vi "General Periodic Sinc.vi"(5 "X":dbl[](array[numeric]), 7 "n":i32, 8 "delta t":dbl, 9 "delay":dbl, 10 "amplitude":dbl, 11 "samples":i32) -> (0 "error":i32, 3 "Periodic Sinc Pattern":dbl[](array[numeric]))   [LabVIEW 2014, in "NI_AALBase.lvlib"]
uses:
  NI_AALBase.lvlib
  lvanlys.dll
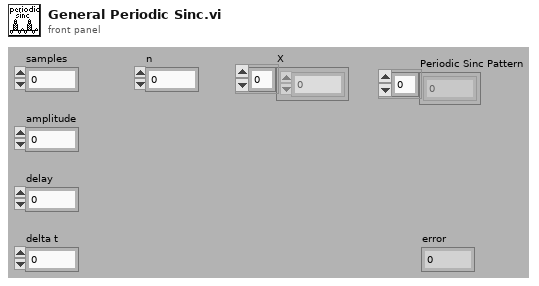
[diagram p1: front panel]
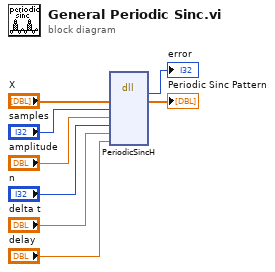
[diagram p0: block diagram]
diagram:
  n1 = dll-call lib="C:/Program Files (x86)/National Instruments/LabVIEW 2014/resource/lvanlys.*" fn="PeriodicSincH"("x"="X", "samples"="samples", "amplitude"="amplitude", "N"="n", "delta t"="delta t", "delay"="delay") -> ("error"=→"error":i32, "x"=→"Periodic Sinc Pattern":dbl[])  [unwired: 8 in, 2 out]
